vi "String_Remove_Extension.vi"(2 "File name with extension":string) -> (0 "Filename without extension":string, 1 "Path & Filename String":string)   [LabVIEW 2017]
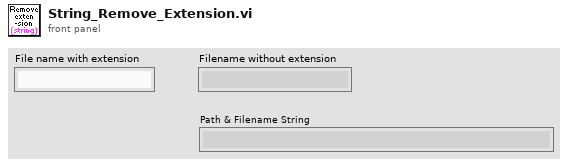
[diagram p1: front panel]
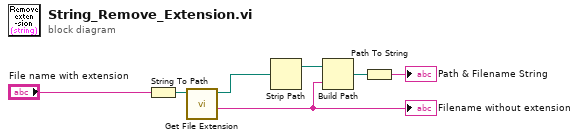
[diagram p0: block diagram]
diagram:
  n1 = String To Path(string="File name with extension") -> (path=w6:path)
  n2 = call <vilib>:"Get File Extension.vi"("file"=w6) -> ("filename without extension"=w3:string, "dup file"=w5:path)  [unwired: 6 in, 3 out]
  "Filename without extension" <- w3
  n3 = Strip Path(path=w5) -> (stripped path=w4:path)  [unwired: 1 out]
  n4 = Build Path(base path=w4, name or relative path=w3) -> (appended path=w2:path)
  n5 = Path To String(path=w2) -> (string=→"Path & Filename String":string)
